vi "WILT.vi"() -> ()   [LabVIEW 2016] (continued)
                n802 = Unbundle By Name(w1538) -> ("Agilent Switches"=w1537:T2[])
                n803 = local read "Test Type"() -> (w1531:T12)
                n804 = Number To Decimal String(number=15) -> (decimal integer string=w1541:string)  [unwired: 1 in]
                n805 = Not(x=w1533) -> (.not. x?=w1540:bool)
                n806 = call "WILT Agilent Valve Control.vi"("Station In"=w1541, "Agilent Channels In"=w1537, "Semaphore"=w1539, "Search"=T19 "Start Button", "Open/Close (F:Close)"=w1540, "error in (no error)"=w1536, "Test Type"=w1531, "Number Of Cycles"=w1530, "Cycle Time (mS)"=w1529) -> ("error out"=w1535:errorcluster)  [unwired: 4 in, 2 out]
              }
            }
            n807 = call <vilib>:"Add State(s) to Queue__jki_lib_state_machine.vi"("State(s) in (\"\")"=w1527) -> ("States Out"=w1526:string)  [unwired: 14 in]
          }
          event Value Change {
            n808 = event-data() -> ("NewVal"=w1542:bool)  [unwired: 1 in, 1 out]
            n809 = local read "Number of ON/OFF Cycles"() -> (w1544:i32)
            n810 = local read "Valve ON Time (mS)"() -> (w1543:u32)
            n811 = local read "Agilent Semaphore"() -> (w1552:T1[])
            n812 = Unbundle By Name(w1551) -> ("Agilent Switches"=w1550:T2[])
            n813 = local read "Test Type"() -> (w1545:T12)
            n814 = Number To Decimal String(number=16) -> (decimal integer string=w1554:string)  [unwired: 1 in]
            n815 = Not(x=w1542) -> (.not. x?=w1553:bool)
            n816 = call "WILT Agilent Valve Control.vi"("Station In"=w1554, "Agilent Channels In"=w1550, "Semaphore"=w1552, "Search"=T19 "Start Button", "Open/Close (F:Close)"=w1553, "error in (no error)"=w1549, "Test Type"=w1545, "Number Of Cycles"=w1544, "Cycle Time (mS)"=w1543) -> ("error out"=w1548:errorcluster)  [unwired: 4 in, 2 out]
            n817 = call <vilib>:"Add State(s) to Queue__jki_lib_state_machine.vi"("State(s) in (\"\")"=w1556) -> ("States Out"=w1555:string)  [unwired: 14 in]
          }
          event Value Change {
            n818 = event-data() -> ("NewVal"=w1557:bool)  [unwired: 1 in, 1 out]
            n819 = case shown="False" w1557 {
              tunnel: w1560 -> [_ w1573]
              tunnel: w1559 -> [w1563 w1571]
              tunnel: [w1563 w1570] -> w1558
              tunnel: w1557 -> [_ w1564]
              frame False {
              }
              frame True {
                n820 = local read "Number of ON/OFF Cycles"() -> (w1566:i32)
                n821 = local read "Valve ON Time (mS)"() -> (w1565:u32)
                n822 = local read "Agilent Semaphore"() -> (w1574:T1[])
                n823 = Unbundle By Name(w1573) -> ("Agilent Switches"=w1572:T2[])
                n824 = local read "Test Type"() -> (w1567:T12)
                n825 = Number To Decimal String(number=17) -> (decimal integer string=w1576:string)  [unwired: 1 in]
                n826 = Not(x=w1564) -> (.not. x?=w1575:bool)
                n827 = call "WILT Agilent Valve Control.vi"("Station In"=w1576, "Agilent Channels In"=w1572, "Semaphore"=w1574, "Search"=T19 "Start Button", "Open/Close (F:Close)"=w1575, "error in (no error)"=w1571, "Test Type"=w1567, "Number Of Cycles"=w1566, "Cycle Time (mS)"=w1565) -> ("error out"=w1570:errorcluster)  [unwired: 4 in, 2 out]
              }
            }
            n828 = call <vilib>:"Add State(s) to Queue__jki_lib_state_machine.vi"("State(s) in (\"\")"=w1562) -> ("States Out"=w1561:string)  [unwired: 14 in]
          }
          event Value Change {
            n829 = event-data() -> ("NewVal"=w1577:bool)  [unwired: 1 in, 1 out]
            n830 = case shown="False" w1577 {
              tunnel: w1580 -> [_ w1593]
              tunnel: w1579 -> [w1583 w1591]
              tunnel: [w1583 w1590] -> w1578
              tunnel: w1577 -> [_ w1584]
              frame False {
              }
              frame True {
                n831 = local read "Number of ON/OFF Cycles"() -> (w1586:i32)
                n832 = local read "Valve ON Time (mS)"() -> (w1585:u32)
                n833 = local read "Agilent Semaphore"() -> (w1594:T1[])
                n834 = Unbundle By Name(w1593) -> ("Agilent Switches"=w1592:T2[])
                n835 = local read "Test Type"() -> (w1587:T12)
                n836 = Number To Decimal String(number=18) -> (decimal integer string=w1596:string)  [unwired: 1 in]
                n837 = Not(x=w1584) -> (.not. x?=w1595:bool)
                n838 = call "WILT Agilent Valve Control.vi"("Station In"=w1596, "Agilent Channels In"=w1592, "Semaphore"=w1594, "Search"=T19 "Start Button", "Open/Close (F:Close)"=w1595, "error in (no error)"=w1591, "Test Type"=w1587, "Number Of Cycles"=w1586, "Cycle Time (mS)"=w1585) -> ("error out"=w1590:errorcluster)  [unwired: 4 in, 2 out]
              }
            }
            n839 = call <vilib>:"Add State(s) to Queue__jki_lib_state_machine.vi"("State(s) in (\"\")"=w1582) -> ("States Out"=w1581:string)  [unwired: 14 in]
          }
          event Value Change {
            n840 = event-data() -> ("NewVal"=w1597:bool)  [unwired: 1 in, 1 out]
            n841 = case shown="False" w1597 {
              tunnel: w1600 -> [_ w1613]
              tunnel: w1599 -> [w1603 w1611]
              tunnel: [w1603 w1610] -> w1598
              tunnel: w1597 -> [_ w1604]
              frame False {
              }
              frame True {
                n842 = local read "Number of ON/OFF Cycles"() -> (w1606:i32)
                n843 = local read "Valve ON Time (mS)"() -> (w1605:u32)
                n844 = local read "Agilent Semaphore"() -> (w1614:T1[])
                n845 = Unbundle By Name(w1613) -> ("Agilent Switches"=w1612:T2[])
                n846 = local read "Test Type"() -> (w1607:T12)
                n847 = Number To Decimal String(number=19) -> (decimal integer string=w1616:string)  [unwired: 1 in]
                n848 = Not(x=w1604) -> (.not. x?=w1615:bool)
                n849 = call "WILT Agilent Valve Control.vi"("Station In"=w1616, "Agilent Channels In"=w1612, "Semaphore"=w1614, "Search"=T19 "Start Button", "Open/Close (F:Close)"=w1615, "error in (no error)"=w1611, "Test Type"=w1607, "Number Of Cycles"=w1606, "Cycle Time (mS)"=w1605) -> ("error out"=w1610:errorcluster)  [unwired: 4 in, 2 out]
              }
            }
            n850 = call <vilib>:"Add State(s) to Queue__jki_lib_state_machine.vi"("State(s) in (\"\")"=w1602) -> ("States Out"=w1601:string)  [unwired: 14 in]
          }
          event Value Change {
            n851 = event-data() -> ("NewVal"=w1617:bool)  [unwired: 1 in, 1 out]
            n852 = case shown="False" w1617 {
              tunnel: w1620 -> [_ w1633]
              tunnel: w1619 -> [w1623 w1631]
              tunnel: [w1623 w1630] -> w1618
              tunnel: w1617 -> [_ w1624]
              frame False {
              }
              frame True {
                n853 = local read "Number of ON/OFF Cycles"() -> (w1626:i32)
                n854 = local read "Valve ON Time (mS)"() -> (w1625:u32)
                n855 = local read "Agilent Semaphore"() -> (w1634:T1[])
                n856 = Unbundle By Name(w1633) -> ("Agilent Switches"=w1632:T2[])
                n857 = local read "Test Type"() -> (w1627:T12)
                n858 = Number To Decimal String(number=20) -> (decimal integer string=w1636:string)  [unwired: 1 in]
                n859 = Not(x=w1624) -> (.not. x?=w1635:bool)
                n860 = call "WILT Agilent Valve Control.vi"("Station In"=w1636, "Agilent Channels In"=w1632, "Semaphore"=w1634, "Search"=T19 "Start Button", "Open/Close (F:Close)"=w1635, "error in (no error)"=w1631, "Test Type"=w1627, "Number Of Cycles"=w1626, "Cycle Time (mS)"=w1625) -> ("error out"=w1630:errorcluster)  [unwired: 4 in, 2 out]
              }
            }
            n861 = call <vilib>:"Add State(s) to Queue__jki_lib_state_machine.vi"("State(s) in (\"\")"=w1622) -> ("States Out"=w1621:string)  [unwired: 14 in]
          }
          event Value Change {
            n862 = event-data() -> ("NewVal"=w1637:bool)  [unwired: 1 in, 1 out]
            n863 = case shown="False" w1637 {
              tunnel: w1640 -> [_ w1653]
              tunnel: w1639 -> [w1643 w1651]
              tunnel: [w1643 w1650] -> w1638
              tunnel: w1637 -> [_ w1644]
              frame False {
              }
              frame True {
                n864 = local read "Number of ON/OFF Cycles"() -> (w1646:i32)
                n865 = local read "Valve ON Time (mS)"() -> (w1645:u32)
                n866 = local read "Agilent Semaphore"() -> (w1654:T1[])
                n867 = Unbundle By Name(w1653) -> ("Agilent Switches"=w1652:T2[])
                n868 = local read "Test Type"() -> (w1647:T12)
                n869 = Number To Decimal String(number=21) -> (decimal integer string=w1656:string)  [unwired: 1 in]
                n870 = Not(x=w1644) -> (.not. x?=w1655:bool)
                n871 = call "WILT Agilent Valve Control.vi"("Station In"=w1656, "Agilent Channels In"=w1652, "Semaphore"=w1654, "Search"=T19 "Start Button", "Open/Close (F:Close)"=w1655, "error in (no error)"=w1651, "Test Type"=w1647, "Number Of Cycles"=w1646, "Cycle Time (mS)"=w1645) -> ("error out"=w1650:errorcluster)  [unwired: 4 in, 2 out]
              }
            }
            n872 = call <vilib>:"Add State(s) to Queue__jki_lib_state_machine.vi"("State(s) in (\"\")"=w1642) -> ("States Out"=w1641:string)  [unwired: 14 in]
          }
          event Value Change {
            n873 = event-data() -> ("NewVal"=w1657:bool)  [unwired: 1 in, 1 out]
            n874 = case shown="False" w1657 {
              tunnel: w1660 -> [_ w1673]
              tunnel: w1659 -> [w1663 w1671]
              tunnel: [w1663 w1670] -> w1658
              tunnel: w1657 -> [_ w1664]
              frame False {
              }
              frame True {
                n875 = local read "Number of ON/OFF Cycles"() -> (w1666:i32)
                n876 = local read "Valve ON Time (mS)"() -> (w1665:u32)
                n877 = local read "Agilent Semaphore"() -> (w1674:T1[])
                n878 = Unbundle By Name(w1673) -> ("Agilent Switches"=w1672:T2[])
                n879 = local read "Test Type"() -> (w1667:T12)
                n880 = Number To Decimal String(number=22) -> (decimal integer string=w1676:string)  [unwired: 1 in]
                n881 = Not(x=w1664) -> (.not. x?=w1675:bool)
                n882 = call "WILT Agilent Valve Control.vi"("Station In"=w1676, "Agilent Channels In"=w1672, "Semaphore"=w1674, "Search"=T19 "Start Button", "Open/Close (F:Close)"=w1675, "error in (no error)"=w1671, "Test Type"=w1667, "Number Of Cycles"=w1666, "Cycle Time (mS)"=w1665) -> ("error out"=w1670:errorcluster)  [unwired: 4 in, 2 out]
              }
            }
            n883 = call <vilib>:"Add State(s) to Queue__jki_lib_state_machine.vi"("State(s) in (\"\")"=w1662) -> ("States Out"=w1661:string)  [unwired: 14 in]
          }
          event Value Change {
            n884 = event-data() -> ("NewVal"=w1677:bool)  [unwired: 1 in, 1 out]
            n885 = case shown="False" w1677 {
              tunnel: w1680 -> [_ w1693]
              tunnel: w1679 -> [w1683 w1691]
              tunnel: [w1683 w1690] -> w1678
              tunnel: w1677 -> [_ w1684]
              frame False {
              }
              frame True {
                n886 = local read "Number of ON/OFF Cycles"() -> (w1686:i32)
                n887 = local read "Valve ON Time (mS)"() -> (w1685:u32)
                n888 = local read "Agilent Semaphore"() -> (w1694:T1[])
                n889 = Unbundle By Name(w1693) -> ("Agilent Switches"=w1692:T2[])
                n890 = local read "Test Type"() -> (w1687:T12)
                n891 = Number To Decimal String(number=23) -> (decimal integer string=w1696:string)  [unwired: 1 in]
                n892 = Not(x=w1684) -> (.not. x?=w1695:bool)
                n893 = call "WILT Agilent Valve Control.vi"("Station In"=w1696, "Agilent Channels In"=w1692, "Semaphore"=w1694, "Search"=T19 "Start Button", "Open/Close (F:Close)"=w1695, "error in (no error)"=w1691, "Test Type"=w1687, "Number Of Cycles"=w1686, "Cycle Time (mS)"=w1685) -> ("error out"=w1690:errorcluster)  [unwired: 4 in, 2 out]
              }
            }
            n894 = call <vilib>:"Add State(s) to Queue__jki_lib_state_machine.vi"("State(s) in (\"\")"=w1682) -> ("States Out"=w1681:string)  [unwired: 14 in]
          }
          event Value Change {
            n895 = event-data() -> ("NewVal"=w1697:bool)  [unwired: 1 in, 1 out]
            n896 = case shown="False" w1697 {
              tunnel: w1700 -> [_ w1713]
              tunnel: w1699 -> [w1703 w1711]
              tunnel: [w1703 w1710] -> w1698
              tunnel: w1697 -> [_ w1704]
              frame False {
              }
              frame True {
                n897 = local read "Number of ON/OFF Cycles"() -> (w1706:i32)
                n898 = local read "Valve ON Time (mS)"() -> (w1705:u32)
                n899 = local read "Agilent Semaphore"() -> (w1714:T1[])
                n900 = Unbundle By Name(w1713) -> ("Agilent Switches"=w1712:T2[])
                n901 = local read "Test Type"() -> (w1707:T12)
                n902 = Number To Decimal String(number=24) -> (decimal integer string=w1716:string)  [unwired: 1 in]
                n903 = Not(x=w1704) -> (.not. x?=w1715:bool)
                n904 = call "WILT Agilent Valve Control.vi"("Station In"=w1716, "Agilent Channels In"=w1712, "Semaphore"=w1714, "Search"=T19 "Start Button", "Open/Close (F:Close)"=w1715, "error in (no error)"=w1711, "Test Type"=w1707, "Number Of Cycles"=w1706, "Cycle Time (mS)"=w1705) -> ("error out"=w1710:errorcluster)  [unwired: 4 in, 2 out]
              }
            }
            n905 = call <vilib>:"Add State(s) to Queue__jki_lib_state_machine.vi"("State(s) in (\"\")"=w1702) -> ("States Out"=w1701:string)  [unwired: 14 in]
          }
          event Value Change {
            n906 = event-data() -> ("NewVal"=w1717:bool)  [unwired: 1 in, 1 out]
            n907 = case shown="False" w1717 {
              tunnel: w1720 -> [_ w1733]
              tunnel: w1719 -> [w1723 w1731]
              tunnel: [w1723 w1730] -> w1718
              tunnel: w1717 -> [_ w1724]
              frame False {
              }
              frame True {
                n908 = local read "Number of ON/OFF Cycles"() -> (w1726:i32)
                n909 = local read "Valve ON Time (mS)"() -> (w1725:u32)
                n910 = local read "Agilent Semaphore"() -> (w1734:T1[])
                n911 = Unbundle By Name(w1733) -> ("Agilent Switches"=w1732:T2[])
                n912 = local read "Test Type"() -> (w1727:T12)
                n913 = Number To Decimal String(number=25) -> (decimal integer string=w1736:string)  [unwired: 1 in]
                n914 = Not(x=w1724) -> (.not. x?=w1735:bool)
                n915 = call "WILT Agilent Valve Control.vi"("Station In"=w1736, "Agilent Channels In"=w1732, "Semaphore"=w1734, "Search"=T19 "Start Button", "Open/Close (F:Close)"=w1735, "error in (no error)"=w1731, "Test Type"=w1727, "Number Of Cycles"=w1726, "Cycle Time (mS)"=w1725) -> ("error out"=w1730:errorcluster)  [unwired: 4 in, 2 out]
              }
            }
            n916 = call <vilib>:"Add State(s) to Queue__jki_lib_state_machine.vi"("State(s) in (\"\")"=w1722) -> ("States Out"=w1721:string)  [unwired: 14 in]
          }
          event Value Change {
            n917 = event-data() -> ("NewVal"=w1737:bool)  [unwired: 1 in, 1 out]
            n918 = case shown="False" w1737 {
              tunnel: w1740 -> [_ w1753]
              tunnel: w1739 -> [w1743 w1751]
              tunnel: [w1743 w1750] -> w1738
              tunnel: w1737 -> [_ w1744]
              frame False {
              }
              frame True {
                n919 = local read "Number of ON/OFF Cycles"() -> (w1746:i32)
                n920 = local read "Valve ON Time (mS)"() -> (w1745:u32)
                n921 = local read "Agilent Semaphore"() -> (w1754:T1[])
                n922 = Unbundle By Name(w1753) -> ("Agilent Switches"=w1752:T2[])
                n923 = local read "Test Type"() -> (w1747:T12)
                n924 = Number To Decimal String(number=26) -> (decimal integer string=w1756:string)  [unwired: 1 in]
                n925 = Not(x=w1744) -> (.not. x?=w1755:bool)
                n926 = call "WILT Agilent Valve Control.vi"("Station In"=w1756, "Agilent Channels In"=w1752, "Semaphore"=w1754, "Search"=T19 "Start Button", "Open/Close (F:Close)"=w1755, "error in (no error)"=w1751, "Test Type"=w1747, "Number Of Cycles"=w1746, "Cycle Time (mS)"=w1745) -> ("error out"=w1750:errorcluster)  [unwired: 4 in, 2 out]
              }
            }
            n927 = call <vilib>:"Add State(s) to Queue__jki_lib_state_machine.vi"("State(s) in (\"\")"=w1742) -> ("States Out"=w1741:string)  [unwired: 14 in]
          }
          event Value Change {
            n928 = event-data() -> ("NewVal"=w1757:bool)  [unwired: 1 in, 1 out]
            n929 = case shown="False" w1757 {
              tunnel: w1760 -> [_ w1773]
              tunnel: w1759 -> [w1763 w1771]
              tunnel: [w1763 w1770] -> w1758
              tunnel: w1757 -> [_ w1764]
              frame False {
              }
              frame True {
                n930 = local read "Number of ON/OFF Cycles"() -> (w1766:i32)
                n931 = local read "Valve ON Time (mS)"() -> (w1765:u32)
                n932 = local read "Agilent Semaphore"() -> (w1774:T1[])
                n933 = Unbundle By Name(w1773) -> ("Agilent Switches"=w1772:T2[])
                n934 = local read "Test Type"() -> (w1767:T12)
                n935 = Number To Decimal String(number=27) -> (decimal integer string=w1776:string)  [unwired: 1 in]
                n936 = Not(x=w1764) -> (.not. x?=w1775:bool)
                n937 = call "WILT Agilent Valve Control.vi"("Station In"=w1776, "Agilent Channels In"=w1772, "Semaphore"=w1774, "Search"=T19 "Start Button", "Open/Close (F:Close)"=w1775, "error in (no error)"=w1771, "Test Type"=w1767, "Number Of Cycles"=w1766, "Cycle Time (mS)"=w1765) -> ("error out"=w1770:errorcluster)  [unwired: 4 in, 2 out]
              }
            }
            n938 = call <vilib>:"Add State(s) to Queue__jki_lib_state_machine.vi"("State(s) in (\"\")"=w1762) -> ("States Out"=w1761:string)  [unwired: 14 in]
          }
          event Value Change {
            n939 = event-data() -> ("NewVal"=w1777:bool)  [unwired: 1 in, 1 out]
            n940 = case shown="False" w1777 {
              tunnel: w1780 -> [_ w1793]
              tunnel: w1779 -> [w1783 w1791]
              tunnel: [w1783 w1790] -> w1778
              tunnel: w1777 -> [_ w1784]
              frame False {
              }
              frame True {
                n941 = local read "Number of ON/OFF Cycles"() -> (w1786:i32)
                n942 = local read "Valve ON Time (mS)"() -> (w1785:u32)
                n943 = local read "Agilent Semaphore"() -> (w1794:T1[])
                n944 = Unbundle By Name(w1793) -> ("Agilent Switches"=w1792:T2[])
                n945 = local read "Test Type"() -> (w1787:T12)
                n946 = Number To Decimal String(number=28) -> (decimal integer string=w1796:string)  [unwired: 1 in]
                n947 = Not(x=w1784) -> (.not. x?=w1795:bool)
                n948 = call "WILT Agilent Valve Control.vi"("Station In"=w1796, "Agilent Channels In"=w1792, "Semaphore"=w1794, "Search"=T19 "Start Button", "Open/Close (F:Close)"=w1795, "error in (no error)"=w1791, "Test Type"=w1787, "Number Of Cycles"=w1786, "Cycle Time (mS)"=w1785) -> ("error out"=w1790:errorcluster)  [unwired: 4 in, 2 out]
              }
            }
            n949 = call <vilib>:"Add State(s) to Queue__jki_lib_state_machine.vi"("State(s) in (\"\")"=w1782) -> ("States Out"=w1781:string)  [unwired: 14 in]
          }
          event Value Change {
            n950 = event-data() -> ("NewVal"=w1797:bool)  [unwired: 1 in, 1 out]
            n951 = case shown="False" w1797 {
              tunnel: w1800 -> [_ w1813]
              tunnel: w1799 -> [w1803 w1811]
              tunnel: [w1803 w1810] -> w1798
              tunnel: w1797 -> [_ w1804]
              frame False {
              }
              frame True {
                n952 = local read "Number of ON/OFF Cycles"() -> (w1806:i32)
                n953 = local read "Valve ON Time (mS)"() -> (w1805:u32)
                n954 = local read "Agilent Semaphore"() -> (w1814:T1[])
                n955 = Unbundle By Name(w1813) -> ("Agilent Switches"=w1812:T2[])
                n956 = local read "Test Type"() -> (w1807:T12)
                n957 = Number To Decimal String(number=29) -> (decimal integer string=w1816:string)  [unwired: 1 in]
                n958 = Not(x=w1804) -> (.not. x?=w1815:bool)
                n959 = call "WILT Agilent Valve Control.vi"("Station In"=w1816, "Agilent Channels In"=w1812, "Semaphore"=w1814, "Search"=T19 "Start Button", "Open/Close (F:Close)"=w1815, "error in (no error)"=w1811, "Test Type"=w1807, "Number Of Cycles"=w1806, "Cycle Time (mS)"=w1805) -> ("error out"=w1810:errorcluster)  [unwired: 4 in, 2 out]
              }
            }
            n960 = call <vilib>:"Add State(s) to Queue__jki_lib_state_machine.vi"("State(s) in (\"\")"=w1802) -> ("States Out"=w1801:string)  [unwired: 14 in]
          }
          event Value Change {
            n961 = event-data() -> ("NewVal"=w1817:bool)  [unwired: 1 in, 1 out]
            n962 = case shown="False" w1817 {
              tunnel: w1820 -> [_ w1833]
              tunnel: w1819 -> [w1823 w1831]
              tunnel: [w1823 w1830] -> w1818
              tunnel: w1817 -> [_ w1824]
              frame False {
              }
              frame True {
                n963 = local read "Number of ON/OFF Cycles"() -> (w1826:i32)
                n964 = local read "Valve ON Time (mS)"() -> (w1825:u32)
                n965 = local read "Agilent Semaphore"() -> (w1834:T1[])
                n966 = Unbundle By Name(w1833) -> ("Agilent Switches"=w1832:T2[])
                n967 = local read "Test Type"() -> (w1827:T12)
                n968 = Number To Decimal String(number=30) -> (decimal integer string=w1836:string)  [unwired: 1 in]
                n969 = Not(x=w1824) -> (.not. x?=w1835:bool)
                n970 = call "WILT Agilent Valve Control.vi"("Station In"=w1836, "Agilent Channels In"=w1832, "Semaphore"=w1834, "Search"=T19 "Start Button", "Open/Close (F:Close)"=w1835, "error in (no error)"=w1831, "Test Type"=w1827, "Number Of Cycles"=w1826, "Cycle Time (mS)"=w1825) -> ("error out"=w1830:errorcluster)  [unwired: 4 in, 2 out]
              }
            }
            n971 = call <vilib>:"Add State(s) to Queue__jki_lib_state_machine.vi"("State(s) in (\"\")"=w1822) -> ("States Out"=w1821:string)  [unwired: 14 in]
          }
          event Value Change {
            n972 = event-data() -> ("NewVal"=w1837:bool)  [unwired: 1 in, 1 out]
            n973 = case shown="False" w1837 {
              tunnel: w1840 -> [_ w1853]
              tunnel: w1839 -> [w1843 w1851]
              tunnel: [w1843 w1850] -> w1838
              tunnel: w1837 -> [_ w1844]
              frame False {
              }
              frame True {
                n974 = local read "Number of ON/OFF Cycles"() -> (w1846:i32)
                n975 = local read "Valve ON Time (mS)"() -> (w1845:u32)
                n976 = local read "Agilent Semaphore"() -> (w1854:T1[])
                n977 = Unbundle By Name(w1853) -> ("Agilent Switches"=w1852:T2[])
                n978 = local read "Test Type"() -> (w1847:T12)
                n979 = Number To Decimal String(number=31) -> (decimal integer string=w1856:string)  [unwired: 1 in]
                n980 = Not(x=w1844) -> (.not. x?=w1855:bool)
                n981 = call "WILT Agilent Valve Control.vi"("Station In"=w1856, "Agilent Channels In"=w1852, "Semaphore"=w1854, "Search"=T19 "Start Button", "Open/Close (F:Close)"=w1855, "error in (no error)"=w1851, "Test Type"=w1847, "Number Of Cycles"=w1846, "Cycle Time (mS)"=w1845) -> ("error out"=w1850:errorcluster)  [unwired: 4 in, 2 out]
              }
            }
            n982 = call <vilib>:"Add State(s) to Queue__jki_lib_state_machine.vi"("State(s) in (\"\")"=w1842) -> ("States Out"=w1841:string)  [unwired: 14 in]
          }
          event Value Change {
            n983 = event-data() -> ("NewVal"=w1857:bool)  [unwired: 1 in, 1 out]
            n984 = case shown="False" w1857 {
              tunnel: w1860 -> [_ w1873]
              tunnel: w1859 -> [w1863 w1871]
              tunnel: [w1863 w1870] -> w1858
              tunnel: w1857 -> [_ w1864]
              frame False {
              }
              frame True {
                n985 = local read "Number of ON/OFF Cycles"() -> (w1866:i32)
                n986 = local read "Valve ON Time (mS)"() -> (w1865:u32)
                n987 = local read "Agilent Semaphore"() -> (w1874:T1[])
                n988 = Unbundle By Name(w1873) -> ("Agilent Switches"=w1872:T2[])
                n989 = local read "Test Type"() -> (w1867:T12)
                n990 = Number To Decimal String(number=32) -> (decimal integer string=w1876:string)  [unwired: 1 in]
                n991 = Not(x=w1864) -> (.not. x?=w1875:bool)
                n992 = call "WILT Agilent Valve Control.vi"("Station In"=w1876, "Agilent Channels In"=w1872, "Semaphore"=w1874, "Search"=T19 "Start Button", "Open/Close (F:Close)"=w1875, "error in (no error)"=w1871, "Test Type"=w1867, "Number Of Cycles"=w1866, "Cycle Time (mS)"=w1865) -> ("error out"=w1870:errorcluster)  [unwired: 4 in, 2 out]
              }
            }
            n993 = call <vilib>:"Add State(s) to Queue__jki_lib_state_machine.vi"("State(s) in (\"\")"=w1862) -> ("States Out"=w1861:string)  [unwired: 14 in]
          }
          event Value Change {
            n994 = event-data() -> ("NewVal"=w1877:bool)  [unwired: 1 in, 1 out]
            n995 = case shown="False" w1877 {
              tunnel: w1880 -> [_ w1893]
              tunnel: w1879 -> [w1883 w1891]
              tunnel: [w1883 w1890] -> w1878
              tunnel: w1877 -> [_ w1884]
              frame False {
              }
              frame True {
                n996 = local read "Number of ON/OFF Cycles"() -> (w1886:i32)
                n997 = local read "Valve ON Time (mS)"() -> (w1885:u32)
                n998 = local read "Agilent Semaphore"() -> (w1894:T1[])
                n999 = Unbundle By Name(w1893) -> ("Agilent Switches"=w1892:T2[])
                n1000 = local read "Test Type"() -> (w1887:T12)
                n1001 = Number To Decimal String(number=33) -> (decimal integer string=w1896:string)  [unwired: 1 in]
                n1002 = Not(x=w1884) -> (.not. x?=w1895:bool)
                n1003 = call "WILT Agilent Valve Control.vi"("Station In"=w1896, "Agilent Channels In"=w1892, "Semaphore"=w1894, "Search"=T19 "Start Button", "Open/Close (F:Close)"=w1895, "error in (no error)"=w1891, "Test Type"=w1887, "Number Of Cycles"=w1886, "Cycle Time (mS)"=w1885) -> ("error out"=w1890:errorcluster)  [unwired: 4 in, 2 out]
              }
            }
            n1004 = call <vilib>:"Add State(s) to Queue__jki_lib_state_machine.vi"("State(s) in (\"\")"=w1882) -> ("States Out"=w1881:string)  [unwired: 14 in]
          }
          event Value Change {
            n1005 = event-data() -> ("NewVal"=w1897:bool)  [unwired: 1 in, 1 out]
            n1006 = case shown="False" w1897 {
              tunnel: w1900 -> [_ w1913]
              tunnel: w1899 -> [w1903 w1911]
              tunnel: [w1903 w1910] -> w1898
              tunnel: w1897 -> [_ w1904]
              frame False {
              }
              frame True {
                n1007 = local read "Number of ON/OFF Cycles"() -> (w1906:i32)
                n1008 = local read "Valve ON Time (mS)"() -> (w1905:u32)
                n1009 = local read "Agilent Semaphore"() -> (w1914:T1[])
                n1010 = Unbundle By Name(w1913) -> ("Agilent Switches"=w1912:T2[])
                n1011 = local read "Test Type"() -> (w1907:T12)
                n1012 = Number To Decimal String(number=34) -> (decimal integer string=w1916:string)  [unwired: 1 in]
                n1013 = Not(x=w1904) -> (.not. x?=w1915:bool)
                n1014 = call "WILT Agilent Valve Control.vi"("Station In"=w1916, "Agilent Channels In"=w1912, "Semaphore"=w1914, "Search"=T19 "Start Button", "Open/Close (F:Close)"=w1915, "error in (no error)"=w1911, "Test Type"=w1907, "Number Of Cycles"=w1906, "Cycle Time (mS)"=w1905) -> ("error out"=w1910:errorcluster)  [unwired: 4 in, 2 out]
              }
            }
            n1015 = call <vilib>:"Add State(s) to Queue__jki_lib_state_machine.vi"("State(s) in (\"\")"=w1902) -> ("States Out"=w1901:string)  [unwired: 14 in]
          }
          event Value Change {
            n1016 = event-data() -> ("NewVal"=w1917:bool)  [unwired: 1 in, 1 out]
            n1017 = case shown="False" w1917 {
              tunnel: w1920 -> [_ w1933]
              tunnel: w1919 -> [w1923 w1931]
              tunnel: [w1923 w1930] -> w1918
              tunnel: w1917 -> [_ w1924]
              frame False {
              }
              frame True {
                n1018 = local read "Number of ON/OFF Cycles"() -> (w1926:i32)
                n1019 = local read "Valve ON Time (mS)"() -> (w1925:u32)
                n1020 = local read "Agilent Semaphore"() -> (w1934:T1[])
                n1021 = Unbundle By Name(w1933) -> ("Agilent Switches"=w1932:T2[])
                n1022 = local read "Test Type"() -> (w1927:T12)
                n1023 = Number To Decimal String(number=35) -> (decimal integer string=w1936:string)  [unwired: 1 in]
                n1024 = Not(x=w1924) -> (.not. x?=w1935:bool)
                n1025 = call "WILT Agilent Valve Control.vi"("Station In"=w1936, "Agilent Channels In"=w1932, "Semaphore"=w1934, "Search"=T19 "Start Button", "Open/Close (F:Close)"=w1935, "error in (no error)"=w1931, "Test Type"=w1927, "Number Of Cycles"=w1926, "Cycle Time (mS)"=w1925) -> ("error out"=w1930:errorcluster)  [unwired: 4 in, 2 out]
              }
            }
            n1026 = call <vilib>:"Add State(s) to Queue__jki_lib_state_machine.vi"("State(s) in (\"\")"=w1922) -> ("States Out"=w1921:string)  [unwired: 14 in]
          }
          event Value Change {
            n1027 = event-data() -> ("NewVal"=w1937:bool)  [unwired: 1 in, 1 out]
            n1028 = case shown="False" w1937 {
              tunnel: w1940 -> [_ w1953]
              tunnel: w1939 -> [w1943 w1951]
              tunnel: [w1943 w1950] -> w1938
              tunnel: w1937 -> [_ w1944]
              frame False {
              }
              frame True {
                n1029 = local read "Number of ON/OFF Cycles"() -> (w1946:i32)
                n1030 = local read "Valve ON Time (mS)"() -> (w1945:u32)
                n1031 = local read "Agilent Semaphore"() -> (w1954:T1[])
                n1032 = Unbundle By Name(w1953) -> ("Agilent Switches"=w1952:T2[])
                n1033 = local read "Test Type"() -> (w1947:T12)
                n1034 = Number To Decimal String(number=36) -> (decimal integer string=w1956:string)  [unwired: 1 in]
                n1035 = Not(x=w1944) -> (.not. x?=w1955:bool)
                n1036 = call "WILT Agilent Valve Control.vi"("Station In"=w1956, "Agilent Channels In"=w1952, "Semaphore"=w1954, "Search"=T19 "Start Button", "Open/Close (F:Close)"=w1955, "error in (no error)"=w1951, "Test Type"=w1947, "Number Of Cycles"=w1946, "Cycle Time (mS)"=w1945) -> ("error out"=w1950:errorcluster)  [unwired: 4 in, 2 out]
              }
            }
            n1037 = call <vilib>:"Add State(s) to Queue__jki_lib_state_machine.vi"("State(s) in (\"\")"=w1942) -> ("States Out"=w1941:string)  [unwired: 14 in]
          }
          event Value Change {
            n1038 = event-data() -> ("NewVal"=w1957:bool)  [unwired: 1 in, 1 out]
            n1039 = case shown="False" w1957 {
              tunnel: w1960 -> [_ w1973]
              tunnel: w1959 -> [w1963 w1971]
              tunnel: [w1963 w1970] -> w1958
              tunnel: w1957 -> [_ w1964]
              frame False {
              }
              frame True {
                n1040 = local read "Number of ON/OFF Cycles"() -> (w1966:i32)
                n1041 = local read "Valve ON Time (mS)"() -> (w1965:u32)
                n1042 = local read "Agilent Semaphore"() -> (w1974:T1[])
                n1043 = Unbundle By Name(w1973) -> ("Agilent Switches"=w1972:T2[])
                n1044 = local read "Test Type"() -> (w1967:T12)
                n1045 = Number To Decimal String(number=37) -> (decimal integer string=w1976:string)  [unwired: 1 in]
                n1046 = Not(x=w1964) -> (.not. x?=w1975:bool)
                n1047 = call "WILT Agilent Valve Control.vi"("Station In"=w1976, "Agilent Channels In"=w1972, "Semaphore"=w1974, "Search"=T19 "Start Button", "Open/Close (F:Close)"=w1975, "error in (no error)"=w1971, "Test Type"=w1967, "Number Of Cycles"=w1966, "Cycle Time (mS)"=w1965) -> ("error out"=w1970:errorcluster)  [unwired: 4 in, 2 out]
              }
            }
            n1048 = call <vilib>:"Add State(s) to Queue__jki_lib_state_machine.vi"("State(s) in (\"\")"=w1962) -> ("States Out"=w1961:string)  [unwired: 14 in]
          }
          event Value Change {
            n1049 = event-data() -> ("NewVal"=w1977:bool)  [unwired: 1 in, 1 out]
            n1050 = case shown="False" w1977 {
              tunnel: w1980 -> [_ w1993]
              tunnel: w1979 -> [w1983 w1991]
              tunnel: [w1983 w1990] -> w1978
              tunnel: w1977 -> [_ w1984]
              frame False {
              }
              frame True {
                n1051 = local read "Number of ON/OFF Cycles"() -> (w1986:i32)
                n1052 = local read "Valve ON Time (mS)"() -> (w1985:u32)
                n1053 = local read "Agilent Semaphore"() -> (w1994:T1[])
                n1054 = Unbundle By Name(w1993) -> ("Agilent Switches"=w1992:T2[])
                n1055 = local read "Test Type"() -> (w1987:T12)
                n1056 = Number To Decimal String(number=38) -> (decimal integer string=w1996:string)  [unwired: 1 in]
                n1057 = Not(x=w1984) -> (.not. x?=w1995:bool)
                n1058 = call "WILT Agilent Valve Control.vi"("Station In"=w1996, "Agilent Channels In"=w1992, "Semaphore"=w1994, "Search"=T19 "Start Button", "Open/Close (F:Close)"=w1995, "error in (no error)"=w1991, "Test Type"=w1987, "Number Of Cycles"=w1986, "Cycle Time (mS)"=w1985) -> ("error out"=w1990:errorcluster)  [unwired: 4 in, 2 out]
              }
            }
            n1059 = call <vilib>:"Add State(s) to Queue__jki_lib_state_machine.vi"("State(s) in (\"\")"=w1982) -> ("States Out"=w1981:string)  [unwired: 14 in]
          }
          event Value Change {
            n1060 = event-data() -> ("NewVal"=w1997:bool)  [unwired: 1 in, 1 out]
            n1061 = case shown="False" w1997 {
              tunnel: w2000 -> [_ w2013]
              tunnel: w1999 -> [w2003 w2011]
              tunnel: [w2003 w2010] -> w1998
              tunnel: w1997 -> [_ w2004]
              frame False {
              }
              frame True {
                n1062 = local read "Number of ON/OFF Cycles"() -> (w2006:i32)
                n1063 = local read "Valve ON Time (mS)"() -> (w2005:u32)
                n1064 = local read "Agilent Semaphore"() -> (w2014:T1[])
                n1065 = Unbundle By Name(w2013) -> ("Agilent Switches"=w2012:T2[])
                n1066 = local read "Test Type"() -> (w2007:T12)
                n1067 = Number To Decimal String(number=39) -> (decimal integer string=w2016:string)  [unwired: 1 in]
                n1068 = Not(x=w2004) -> (.not. x?=w2015:bool)
                n1069 = call "WILT Agilent Valve Control.vi"("Station In"=w2016, "Agilent Channels In"=w2012, "Semaphore"=w2014, "Search"=T19 "Start Button", "Open/Close (F:Close)"=w2015, "error in (no error)"=w2011, "Test Type"=w2007, "Number Of Cycles"=w2006, "Cycle Time (mS)"=w2005) -> ("error out"=w2010:errorcluster)  [unwired: 4 in, 2 out]
              }
            }
            n1070 = call <vilib>:"Add State(s) to Queue__jki_lib_state_machine.vi"("State(s) in (\"\")"=w2002) -> ("States Out"=w2001:string)  [unwired: 14 in]
          }
          event Value Change {
            n1071 = event-data() -> ("NewVal"=w2017:bool)  [unwired: 1 in, 1 out]
            n1072 = case shown="False" w2017 {
              tunnel: w2020 -> [_ w2033]
              tunnel: w2019 -> [w2023 w2031]
              tunnel: [w2023 w2030] -> w2018
              tunnel: w2017 -> [_ w2024]
              frame False {
              }
              frame True {
                n1073 = local read "Number of ON/OFF Cycles"() -> (w2026:i32)
                n1074 = local read "Valve ON Time (mS)"() -> (w2025:u32)
                n1075 = local read "Agilent Semaphore"() -> (w2034:T1[])
                n1076 = Unbundle By Name(w2033) -> ("Agilent Switches"=w2032:T2[])
                n1077 = local read "Test Type"() -> (w2027:T12)
                n1078 = Number To Decimal String(number=40) -> (decimal integer string=w2036:string)  [unwired: 1 in]
                n1079 = Not(x=w2024) -> (.not. x?=w2035:bool)
                n1080 = call "WILT Agilent Valve Control.vi"("Station In"=w2036, "Agilent Channels In"=w2032, "Semaphore"=w2034, "Search"=T19 "Start Button", "Open/Close (F:Close)"=w2035, "error in (no error)"=w2031, "Test Type"=w2027, "Number Of Cycles"=w2026, "Cycle Time (mS)"=w2025) -> ("error out"=w2030:errorcluster)  [unwired: 4 in, 2 out]
              }
            }
            n1081 = call <vilib>:"Add State(s) to Queue__jki_lib_state_machine.vi"("State(s) in (\"\")"=w2022) -> ("States Out"=w2021:string)  [unwired: 14 in]
          }
          event Value Change {
            n1082 = event-data() -> ("NewVal"=w2037:bool)  [unwired: 1 in, 1 out]
            n1083 = case shown="False" w2037 {
              tunnel: w2040 -> [_ w2053]
              tunnel: w2039 -> [w2043 w2051]
              tunnel: [w2043 w2050] -> w2038
              tunnel: w2037 -> [_ w2044]
              frame False {
              }
              frame True {
                n1084 = local read "Number of ON/OFF Cycles"() -> (w2046:i32)
                n1085 = local read "Valve ON Time (mS)"() -> (w2045:u32)
                n1086 = local read "Agilent Semaphore"() -> (w2054:T1[])
                n1087 = Unbundle By Name(w2053) -> ("Agilent Switches"=w2052:T2[])
                n1088 = local read "Test Type"() -> (w2047:T12)
                n1089 = Number To Decimal String(number=41) -> (decimal integer string=w2056:string)  [unwired: 1 in]
                n1090 = Not(x=w2044) -> (.not. x?=w2055:bool)
                n1091 = call "WILT Agilent Valve Control.vi"("Station In"=w2056, "Agilent Channels In"=w2052, "Semaphore"=w2054, "Search"=T19 "Start Button", "Open/Close (F:Close)"=w2055, "error in (no error)"=w2051, "Test Type"=w2047, "Number Of Cycles"=w2046, "Cycle Time (mS)"=w2045) -> ("error out"=w2050:errorcluster)  [unwired: 4 in, 2 out]
              }
            }
            n1092 = call <vilib>:"Add State(s) to Queue__jki_lib_state_machine.vi"("State(s) in (\"\")"=w2042) -> ("States Out"=w2041:string)  [unwired: 14 in]
          }
          event Value Change {
            n1093 = event-data() -> ("NewVal"=w2057:bool)  [unwired: 1 in, 1 out]
            n1094 = case shown="False" w2057 {
              tunnel: w2060 -> [_ w2073]
              tunnel: w2059 -> [w2063 w2071]
              tunnel: [w2063 w2070] -> w2058
              tunnel: w2057 -> [_ w2064]
              frame False {
              }
              frame True {
                n1095 = local read "Number of ON/OFF Cycles"() -> (w2066:i32)
                n1096 = local read "Valve ON Time (mS)"() -> (w2065:u32)
                n1097 = local read "Agilent Semaphore"() -> (w2074:T1[])
                n1098 = Unbundle By Name(w2073) -> ("Agilent Switches"=w2072:T2[])
                n1099 = local read "Test Type"() -> (w2067:T12)
                n1100 = Number To Decimal String(number=42) -> (decimal integer string=w2076:string)  [unwired: 1 in]
                n1101 = Not(x=w2064) -> (.not. x?=w2075:bool)
                n1102 = call "WILT Agilent Valve Control.vi"("Station In"=w2076, "Agilent Channels In"=w2072, "Semaphore"=w2074, "Search"=T19 "Start Button", "Open/Close (F:Close)"=w2075, "error in (no error)"=w2071, "Test Type"=w2067, "Number Of Cycles"=w2066, "Cycle Time (mS)"=w2065) -> ("error out"=w2070:errorcluster)  [unwired: 4 in, 2 out]
              }
            }
            n1103 = call <vilib>:"Add State(s) to Queue__jki_lib_state_machine.vi"("State(s) in (\"\")"=w2062) -> ("States Out"=w2061:string)  [unwired: 14 in]
          }
          event Value Change {
            n1104 = event-data() -> ("NewVal"=w2077:bool)  [unwired: 1 in, 1 out]
            n1105 = case shown="False" w2077 {
              tunnel: w2080 -> [_ w2093]
              tunnel: w2079 -> [w2083 w2091]
              tunnel: [w2083 w2090] -> w2078
              tunnel: w2077 -> [_ w2084]
              frame False {
              }
              frame True {
                n1106 = local read "Number of ON/OFF Cycles"() -> (w2086:i32)
                n1107 = local read "Valve ON Time (mS)"() -> (w2085:u32)
                n1108 = local read "Agilent Semaphore"() -> (w2094:T1[])
                n1109 = Unbundle By Name(w2093) -> ("Agilent Switches"=w2092:T2[])
                n1110 = local read "Test Type"() -> (w2087:T12)
                n1111 = Number To Decimal String(number=43) -> (decimal integer string=w2096:string)  [unwired: 1 in]
                n1112 = Not(x=w2084) -> (.not. x?=w2095:bool)
                n1113 = call "WILT Agilent Valve Control.vi"("Station In"=w2096, "Agilent Channels In"=w2092, "Semaphore"=w2094, "Search"=T19 "Start Button", "Open/Close (F:Close)"=w2095, "error in (no error)"=w2091, "Test Type"=w2087, "Number Of Cycles"=w2086, "Cycle Time (mS)"=w2085) -> ("error out"=w2090:errorcluster)  [unwired: 4 in, 2 out]
              }
            }
            n1114 = call <vilib>:"Add State(s) to Queue__jki_lib_state_machine.vi"("State(s) in (\"\")"=w2082) -> ("States Out"=w2081:string)  [unwired: 14 in]
          }
          event Value Change {
            n1115 = event-data() -> ("NewVal"=w2097:bool)  [unwired: 1 in, 1 out]
            n1116 = case shown="False" w2097 {
              tunnel: w2100 -> [_ w2113]
              tunnel: w2099 -> [w2103 w2111]
              tunnel: [w2103 w2110] -> w2098
              tunnel: w2097 -> [_ w2104]
              frame False {
              }
              frame True {
                n1117 = local read "Number of ON/OFF Cycles"() -> (w2106:i32)
                n1118 = local read "Valve ON Time (mS)"() -> (w2105:u32)
                n1119 = local read "Agilent Semaphore"() -> (w2114:T1[])
                n1120 = Unbundle By Name(w2113) -> ("Agilent Switches"=w2112:T2[])
                n1121 = local read "Test Type"() -> (w2107:T12)
                n1122 = Number To Decimal String(number=44) -> (decimal integer string=w2116:string)  [unwired: 1 in]
                n1123 = Not(x=w2104) -> (.not. x?=w2115:bool)
                n1124 = call "WILT Agilent Valve Control.vi"("Station In"=w2116, "Agilent Channels In"=w2112, "Semaphore"=w2114, "Search"=T19 "Start Button", "Open/Close (F:Close)"=w2115, "error in (no error)"=w2111, "Test Type"=w2107, "Number Of Cycles"=w2106, "Cycle Time (mS)"=w2105) -> ("error out"=w2110:errorcluster)  [unwired: 4 in, 2 out]
              }
            }
            n1125 = call <vilib>:"Add State(s) to Queue__jki_lib_state_machine.vi"("State(s) in (\"\")"=w2102) -> ("States Out"=w2101:string)  [unwired: 14 in]
          }
          event Value Change {
            n1126 = event-data() -> ("NewVal"=w2117:bool)  [unwired: 1 in, 1 out]
            n1127 = case shown="False" w2117 {
              tunnel: w2120 -> [_ w2133]
              tunnel: w2119 -> [w2123 w2131]
              tunnel: [w2123 w2130] -> w2118
              tunnel: w2117 -> [_ w2124]
              frame False {
              }
              frame True {
                n1128 = local read "Number of ON/OFF Cycles"() -> (w2126:i32)
                n1129 = local read "Valve ON Time (mS)"() -> (w2125:u32)
                n1130 = local read "Agilent Semaphore"() -> (w2134:T1[])
                n1131 = Unbundle By Name(w2133) -> ("Agilent Switches"=w2132:T2[])
                n1132 = local read "Test Type"() -> (w2127:T12)
                n1133 = Number To Decimal String(number=45) -> (decimal integer string=w2136:string)  [unwired: 1 in]
                n1134 = Not(x=w2124) -> (.not. x?=w2135:bool)
                n1135 = call "WILT Agilent Valve Control.vi"("Station In"=w2136, "Agilent Channels In"=w2132, "Semaphore"=w2134, "Search"=T19 "Start Button", "Open/Close (F:Close)"=w2135, "error in (no error)"=w2131, "Test Type"=w2127, "Number Of Cycles"=w2126, "Cycle Time (mS)"=w2125) -> ("error out"=w2130:errorcluster)  [unwired: 4 in, 2 out]
              }
            }
            n1136 = call <vilib>:"Add State(s) to Queue__jki_lib_state_machine.vi"("State(s) in (\"\")"=w2122) -> ("States Out"=w2121:string)  [unwired: 14 in]
          }
          event Value Change {
            n1137 = event-data() -> ("NewVal"=w2137:bool)  [unwired: 1 in, 1 out]
            n1138 = case shown="False" w2137 {
              tunnel: w2140 -> [_ w2153]
              tunnel: w2139 -> [w2143 w2151]
              tunnel: [w2143 w2150] -> w2138
              tunnel: w2137 -> [_ w2144]
              frame False {
              }
              frame True {
                n1139 = local read "Number of ON/OFF Cycles"() -> (w2146:i32)
                n1140 = local read "Valve ON Time (mS)"() -> (w2145:u32)
                n1141 = local read "Agilent Semaphore"() -> (w2154:T1[])
                n1142 = Unbundle By Name(w2153) -> ("Agilent Switches"=w2152:T2[])
                n1143 = local read "Test Type"() -> (w2147:T12)
                n1144 = Number To Decimal String(number=46) -> (decimal integer string=w2156:string)  [unwired: 1 in]
                n1145 = Not(x=w2144) -> (.not. x?=w2155:bool)
                n1146 = call "WILT Agilent Valve Control.vi"("Station In"=w2156, "Agilent Channels In"=w2152, "Semaphore"=w2154, "Search"=T19 "Start Button", "Open/Close (F:Close)"=w2155, "error in (no error)"=w2151, "Test Type"=w2147, "Number Of Cycles"=w2146, "Cycle Time (mS)"=w2145) -> ("error out"=w2150:errorcluster)  [unwired: 4 in, 2 out]
              }
            }
            n1147 = call <vilib>:"Add State(s) to Queue__jki_lib_state_machine.vi"("State(s) in (\"\")"=w2142) -> ("States Out"=w2141:string)  [unwired: 14 in]
          }
          event Value Change {
            n1148 = event-data() -> ("NewVal"=w2157:bool)  [unwired: 1 in, 1 out]
            n1149 = case shown="False" w2157 {
              tunnel: w2160 -> [_ w2173]
              tunnel: w2159 -> [w2163 w2171]
              tunnel: [w2163 w2170] -> w2158
              tunnel: w2157 -> [_ w2164]
              frame False {
              }
              frame True {
                n1150 = local read "Number of ON/OFF Cycles"() -> (w2166:i32)
                n1151 = local read "Valve ON Time (mS)"() -> (w2165:u32)
                n1152 = local read "Agilent Semaphore"() -> (w2174:T1[])
                n1153 = Unbundle By Name(w2173) -> ("Agilent Switches"=w2172:T2[])
                n1154 = local read "Test Type"() -> (w2167:T12)
                n1155 = Number To Decimal String(number=47) -> (decimal integer string=w2176:string)  [unwired: 1 in]
                n1156 = Not(x=w2164) -> (.not. x?=w2175:bool)
                n1157 = call "WILT Agilent Valve Control.vi"("Station In"=w2176, "Agilent Channels In"=w2172, "Semaphore"=w2174, "Search"=T19 "Start Button", "Open/Close (F:Close)"=w2175, "error in (no error)"=w2171, "Test Type"=w2167, "Number Of Cycles"=w2166, "Cycle Time (mS)"=w2165) -> ("error out"=w2170:errorcluster)  [unwired: 4 in, 2 out]
              }
            }
            n1158 = call <vilib>:"Add State(s) to Queue__jki_lib_state_machine.vi"("State(s) in (\"\")"=w2162) -> ("States Out"=w2161:string)  [unwired: 14 in]
          }
          event Value Change {
            n1159 = event-data() -> ("NewVal"=w2177:bool)  [unwired: 1 in, 1 out]
            n1160 = case shown="False" w2177 {
              tunnel: w2180 -> [_ w2193]
              tunnel: w2179 -> [w2183 w2191]
              tunnel: [w2183 w2190] -> w2178
              tunnel: w2177 -> [_ w2184]
              frame False {
              }
              frame True {
                n1161 = local read "Number of ON/OFF Cycles"() -> (w2186:i32)
                n1162 = local read "Valve ON Time (mS)"() -> (w2185:u32)
                n1163 = local read "Agilent Semaphore"() -> (w2194:T1[])
                n1164 = Unbundle By Name(w2193) -> ("Agilent Switches"=w2192:T2[])
                n1165 = local read "Test Type"() -> (w2187:T12)
                n1166 = Number To Decimal String(number=48) -> (decimal integer string=w2196:string)  [unwired: 1 in]
                n1167 = Not(x=w2184) -> (.not. x?=w2195:bool)
                n1168 = call "WILT Agilent Valve Control.vi"("Station In"=w2196, "Agilent Channels In"=w2192, "Semaphore"=w2194, "Search"=T19 "Start Button", "Open/Close (F:Close)"=w2195, "error in (no error)"=w2191, "Test Type"=w2187, "Number Of Cycles"=w2186, "Cycle Time (mS)"=w2185) -> ("error out"=w2190:errorcluster)  [unwired: 4 in, 2 out]
              }
            }
            n1169 = call <vilib>:"Add State(s) to Queue__jki_lib_state_machine.vi"("State(s) in (\"\")"=w2182) -> ("States Out"=w2181:string)  [unwired: 14 in]
          }
          event Value Change {
            n1170 = event-data() -> ("NewVal"=w2197:bool)  [unwired: 1 in, 1 out]
            n1171 = case shown="False" w2197 {
              tunnel: w2200 -> [_ w2213]
              tunnel: w2199 -> [w2203 w2211]
              tunnel: [w2203 w2210] -> w2198
              tunnel: w2197 -> [_ w2204]
              frame False {
              }
              frame True {
                n1172 = local read "Number of ON/OFF Cycles"() -> (w2206:i32)
                n1173 = local read "Valve ON Time (mS)"() -> (w2205:u32)
                n1174 = local read "Agilent Semaphore"() -> (w2214:T1[])
                n1175 = Unbundle By Name(w2213) -> ("Agilent Switches"=w2212:T2[])
                n1176 = local read "Test Type"() -> (w2207:T12)
                n1177 = Number To Decimal String(number=49) -> (decimal integer string=w2216:string)  [unwired: 1 in]
                n1178 = Not(x=w2204) -> (.not. x?=w2215:bool)
                n1179 = call "WILT Agilent Valve Control.vi"("Station In"=w2216, "Agilent Channels In"=w2212, "Semaphore"=w2214, "Search"=T19 "Start Button", "Open/Close (F:Close)"=w2215, "error in (no error)"=w2211, "Test Type"=w2207, "Number Of Cycles"=w2206, "Cycle Time (mS)"=w2205) -> ("error out"=w2210:errorcluster)  [unwired: 4 in, 2 out]
              }
            }
            n1180 = call <vilib>:"Add State(s) to Queue__jki_lib_state_machine.vi"("State(s) in (\"\")"=w2202) -> ("States Out"=w2201:string)  [unwired: 14 in]
          }
          event Value Change {
            n1181 = event-data() -> ("NewVal"=w2217:bool)  [unwired: 1 in, 1 out]
            n1182 = case shown="False" w2217 {
              tunnel: w2220 -> [_ w2233]
              tunnel: w2219 -> [w2223 w2231]
              tunnel: [w2223 w2230] -> w2218
              tunnel: w2217 -> [_ w2224]
              frame False {
              }
              frame True {
                n1183 = local read "Number of ON/OFF Cycles"() -> (w2226:i32)
                n1184 = local read "Valve ON Time (mS)"() -> (w2225:u32)
                n1185 = local read "Agilent Semaphore"() -> (w2234:T1[])
                n1186 = Unbundle By Name(w2233) -> ("Agilent Switches"=w2232:T2[])
                n1187 = local read "Test Type"() -> (w2227:T12)
                n1188 = Number To Decimal String(number=50) -> (decimal integer string=w2236:string)  [unwired: 1 in]
                n1189 = Not(x=w2224) -> (.not. x?=w2235:bool)
                n1190 = call "WILT Agilent Valve Control.vi"("Station In"=w2236, "Agilent Channels In"=w2232, "Semaphore"=w2234, "Search"=T19 "Start Button", "Open/Close (F:Close)"=w2235, "error in (no error)"=w2231, "Test Type"=w2227, "Number Of Cycles"=w2226, "Cycle Time (mS)"=w2225) -> ("error out"=w2230:errorcluster)  [unwired: 4 in, 2 out]
              }
            }
            n1191 = call <vilib>:"Add State(s) to Queue__jki_lib_state_machine.vi"("State(s) in (\"\")"=w2222) -> ("States Out"=w2221:string)  [unwired: 14 in]
          }
          event Value Change {
            n1192 = event-data() -> ("NewVal"=w2237:bool)  [unwired: 1 in, 1 out]
            n1193 = case shown="False" w2237 {
              tunnel: w2240 -> [_ w2253]
              tunnel: w2239 -> [w2243 w2251]
              tunnel: [w2243 w2250] -> w2238
              tunnel: w2237 -> [_ w2244]
              frame False {
              }
              frame True {
                n1194 = local read "Number of ON/OFF Cycles"() -> (w2246:i32)
                n1195 = local read "Valve ON Time (mS)"() -> (w2245:u32)
                n1196 = local read "Agilent Semaphore"() -> (w2254:T1[])
                n1197 = Unbundle By Name(w2253) -> ("Agilent Switches"=w2252:T2[])
                n1198 = local read "Test Type"() -> (w2247:T12)
                n1199 = Number To Decimal String(number=51) -> (decimal integer string=w2256:string)  [unwired: 1 in]
                n1200 = Not(x=w2244) -> (.not. x?=w2255:bool)
                n1201 = call "WILT Agilent Valve Control.vi"("Station In"=w2256, "Agilent Channels In"=w2252, "Semaphore"=w2254, "Search"=T19 "Start Button", "Open/Close (F:Close)"=w2255, "error in (no error)"=w2251, "Test Type"=w2247, "Number Of Cycles"=w2246, "Cycle Time (mS)"=w2245) -> ("error out"=w2250:errorcluster)  [unwired: 4 in, 2 out]
              }
            }
            n1202 = call <vilib>:"Add State(s) to Queue__jki_lib_state_machine.vi"("State(s) in (\"\")"=w2242) -> ("States Out"=w2241:string)  [unwired: 14 in]
          }
          event Value Change {
            n1203 = event-data() -> ("NewVal"=w2257:bool)  [unwired: 1 in, 1 out]
            n1204 = case shown="True" w2257 {
              tunnel: w2260 -> [_ w2273]
              tunnel: w2259 -> [w2263 w2271]
              tunnel: [w2263 w2270] -> w2258
              tunnel: w2257 -> [_ w2264]
              frame False {
              }
              frame True {
                n1205 = local read "Number of ON/OFF Cycles"() -> (w2266:i32)
                n1206 = local read "Valve ON Time (mS)"() -> (w2265:u32)
                n1207 = local read "Agilent Semaphore"() -> (w2274:T1[])
                n1208 = Unbundle By Name(w2273) -> ("Agilent Switches"=w2272:T2[])
                n1209 = local read "Test Type"() -> (w2267:T12)
                n1210 = Number To Decimal String(number=52) -> (decimal integer string=w2276:string)  [unwired: 1 in]
                n1211 = Not(x=w2264) -> (.not. x?=w2275:bool)
                n1212 = call "WILT Agilent Valve Control.vi"("Station In"=w2276, "Agilent Channels In"=w2272, "Semaphore"=w2274, "Search"=T19 "Start Button", "Open/Close (F:Close)"=w2275, "error in (no error)"=w2271, "Test Type"=w2267, "Number Of Cycles"=w2266, "Cycle Time (mS)"=w2265) -> ("error out"=w2270:errorcluster)  [unwired: 4 in, 2 out]
              }
            }
            n1213 = call <vilib>:"Add State(s) to Queue__jki_lib_state_machine.vi"("State(s) in (\"\")"=w2262) -> ("States Out"=w2261:string)  [unwired: 14 in]
          }
          event Value Change {
            n1214 = event-data() -> ("NewVal"=w2277:bool)  [unwired: 1 in, 1 out]
            n1215 = case shown="True" w2277 {
              tunnel: w2280 -> [_ w2293]
              tunnel: w2279 -> [w2283 w2291]
              tunnel: [w2283 w2290] -> w2278
              tunnel: w2277 -> [_ w2284]
              frame False {
              }
              frame True {
                n1216 = local read "Number of ON/OFF Cycles"() -> (w2286:i32)
                n1217 = local read "Valve ON Time (mS)"() -> (w2285:u32)
                n1218 = local read "Agilent Semaphore"() -> (w2294:T1[])
                n1219 = Unbundle By Name(w2293) -> ("Agilent Switches"=w2292:T2[])
                n1220 = local read "Test Type"() -> (w2287:T12)
                n1221 = Number To Decimal String(number=53) -> (decimal integer string=w2296:string)  [unwired: 1 in]
                n1222 = Not(x=w2284) -> (.not. x?=w2295:bool)
                n1223 = call "WILT Agilent Valve Control.vi"("Station In"=w2296, "Agilent Channels In"=w2292, "Semaphore"=w2294, "Search"=T19 "Start Button", "Open/Close (F:Close)"=w2295, "error in (no error)"=w2291, "Test Type"=w2287, "Number Of Cycles"=w2286, "Cycle Time (mS)"=w2285) -> ("error out"=w2290:errorcluster)  [unwired: 4 in, 2 out]
              }
            }
            n1224 = call <vilib>:"Add State(s) to Queue__jki_lib_state_machine.vi"("State(s) in (\"\")"=w2282) -> ("States Out"=w2281:string)  [unwired: 14 in]
          }
          event Value Change {
            n1225 = event-data() -> ("NewVal"=w2297:bool)  [unwired: 1 in, 1 out]
            n1226 = case shown="False" w2297 {
              tunnel: w2300 -> [_ w2313]
              tunnel: w2299 -> [w2303 w2311]
              tunnel: [w2303 w2310] -> w2298
              tunnel: w2297 -> [_ w2304]
              frame False {
              }
              frame True {
                n1227 = local read "Number of ON/OFF Cycles"() -> (w2306:i32)
                n1228 = local read "Valve ON Time (mS)"() -> (w2305:u32)
                n1229 = local read "Agilent Semaphore"() -> (w2314:T1[])
                n1230 = Unbundle By Name(w2313) -> ("Agilent Switches"=w2312:T2[])
                n1231 = local read "Test Type"() -> (w2307:T12)
                n1232 = Number To Decimal String(number=54) -> (decimal integer string=w2316:string)  [unwired: 1 in]
